vi "Trial v4.vi"(2 "error in (no error)":errorcluster, 3 "queue in":refnum<queue>, 4 "DDA":bool=TRUE) -> (0 "error out":errorcluster, 1 "queue out":refnum<queue>)   [LabVIEW 2017]
uses:
  SubVI/Global.vi
  <vilib>/Analysis/NI_AALPro.lvlib
  <vilib>/robotics/Kinematics/NI_Kinematics.lvlib
  Control/RPY.ctl
  Control/Damping.ctl
  <vilib>/Analysis/NI_AALBase.lvlib
  <vilib>/Analysis/baseanly.llb/Real Dot Product.vi
  <vilib>/Analysis/_algsub.llb/Real Vector Norm.vi
panel:
  in  "RoM (deg)":dbl=75.0 format="%#_13g"
  in  "Weber's Rule":dbl[](array[numeric])=[1.05, 1.0, 0.95]
  in  "n x(s, a)":i32=3
  in  "n x(s)":i32=3
  in  "Variable":T1
  in  "Time Target (s)":dbl=10.0
  in  "epsilon":dbl=0.1
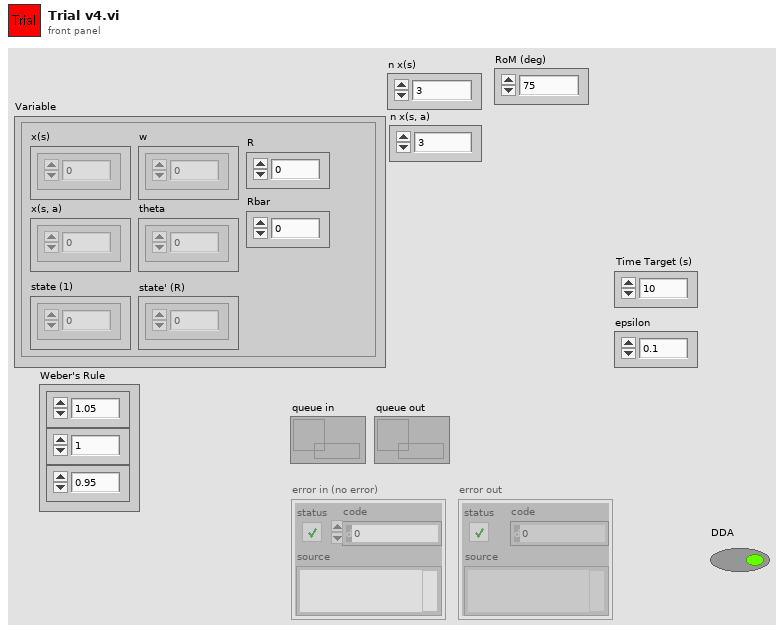
[diagram p1: front panel]
types:
  T1 = cluster{"x(s)":dbl[], "x(s, a)":dbl[], "w":dbl[], "theta":dbl[], "state (1)":dbl[], "state' (R)":dbl[], "R":dbl, "Rbar":dbl}
  T2 = typedef "RPY.ctl" = cluster{"roll":dbl, "pitch":dbl, "yaw":dbl}
  T3 = typedef "NI_Matrix.lvlib/RealMatrix.ctl" = dbl[][]
  T4 = typedef "Damping.ctl" = cluster{"Cx":dbl, "Cy":dbl, "Cz":dbl}
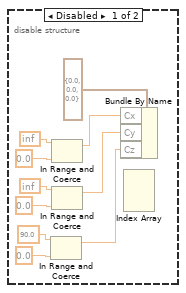
[diagram p2: hidden frame]
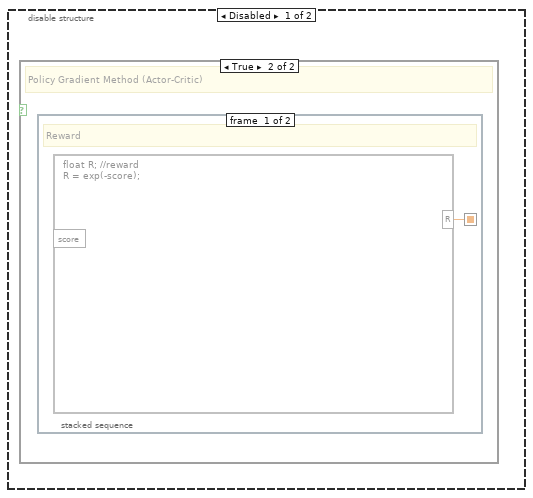
[diagram p3: hidden frame]
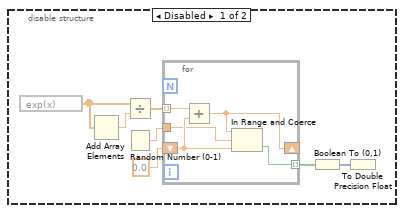
[diagram p6: hidden frame]
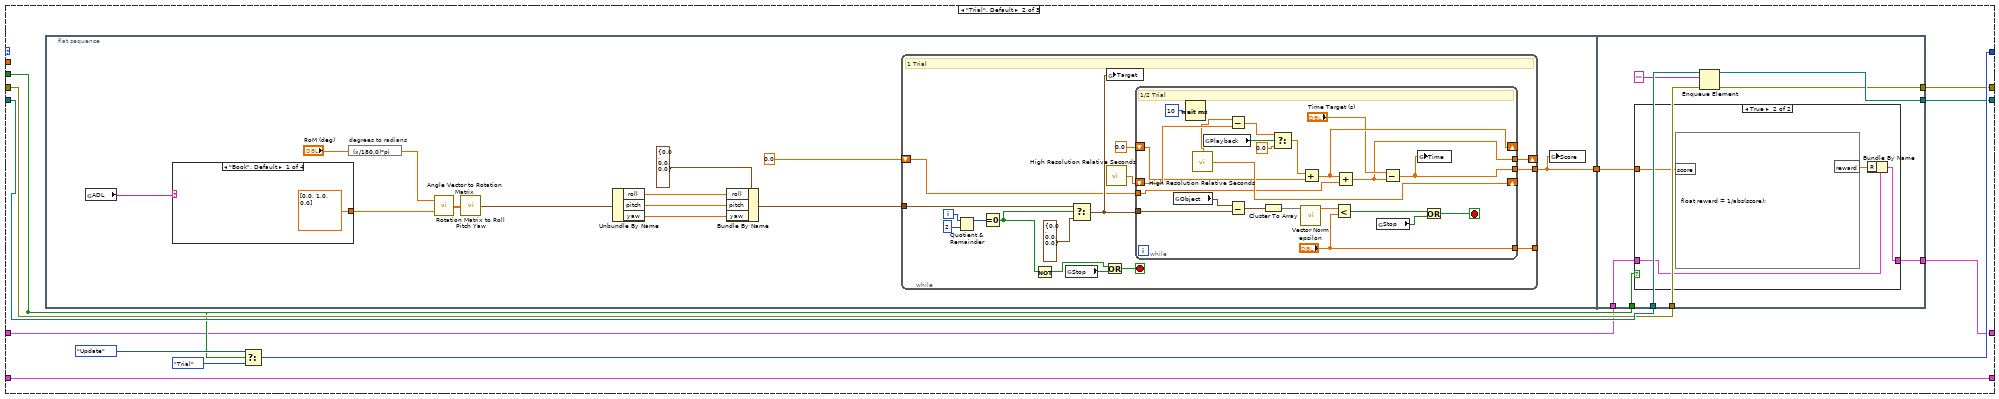
[diagram p7: hidden frame]
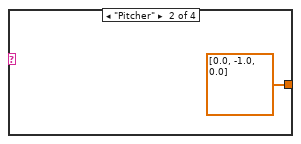
[diagram p8: hidden frame]
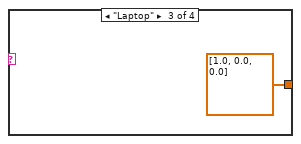
[diagram p9: hidden frame]
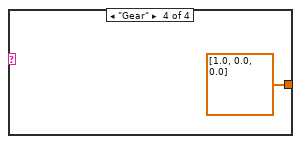
[diagram p10: hidden frame]
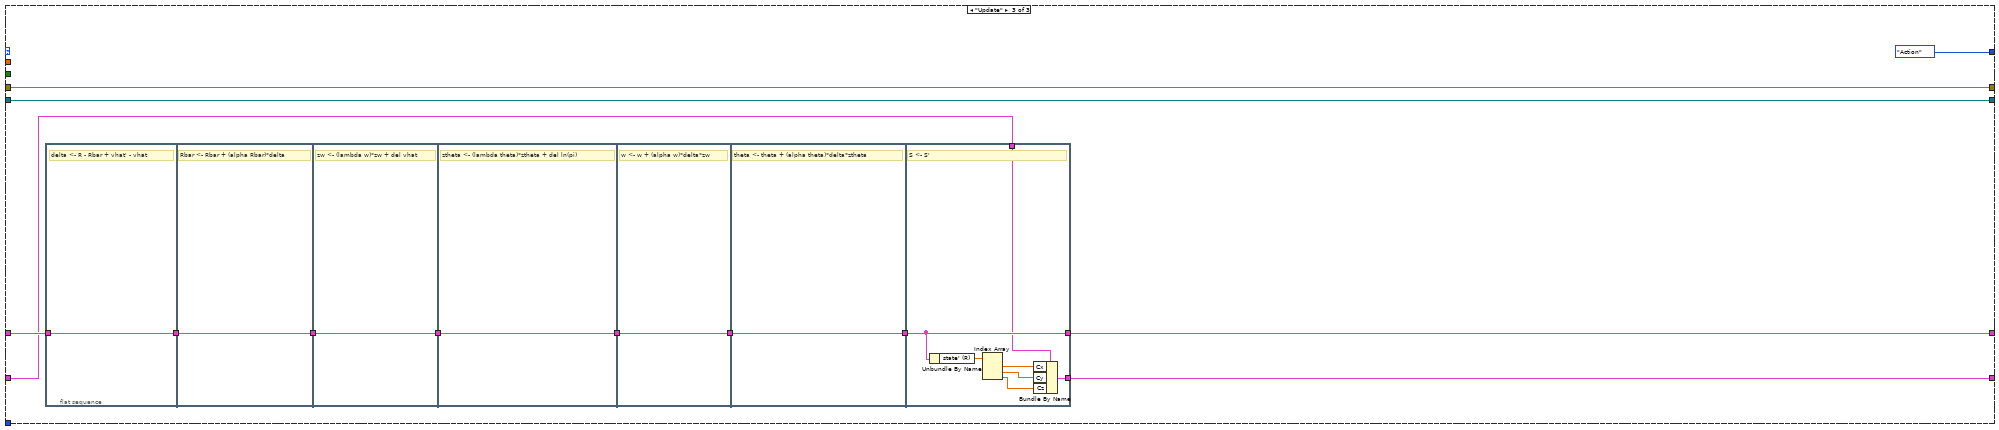
[diagram p12: hidden frame]
diagram:
  n1 = flat-sequence {
    tunnel: "error in (no error)" -> [w15]
    tunnel: "queue in" -> [w17]
    tunnel: "DDA" -> [w10]
    tunnel: [w16] -> w2
    tunnel: [w14] -> w1
    frame #0 {
      n2 = flat-sequence {
        tunnel: [w34] -> w8
        tunnel: ["n x(s, a)"] -> w7
        tunnel: [w31] -> w6
        frame #0 {
          w32 = 3
          n3 = for {
            N: w32 -> [_]
            tunnel: [w37] -> w31 mode=concatenating
            tunnel: w32 -> [w36]
            tunnel: w32 -> [w35]
            i -> [w38]
            n4 = for {
              N: w36 -> [_]
              tunnel: w38 -> [w42]
              tunnel: [w40] -> w37 mode=concatenating
              tunnel: w35 -> [w39]
              i -> [w41]
              n5 = for {
                N: w39 -> [_]
                tunnel: w42 -> [w49]
                tunnel: w41 -> [w48]
                tunnel: [w43] -> w40 mode=indexing
                i -> [w47]
                n6 = Index Array(array="Weber's Rule", index #1=w49, index #2=w48, index #3=w47) -> (element #1=w46:dbl, element #2=w45:dbl, element #3=w44:dbl)
                n7 = Build Array(w46, w45, w44) -> (w43:dbl[])
              }
            }
          }
          n8 = call "Feature Vector State Action.vi"("n x(s, a)"="n x(s, a)", "action"=0.0, "state"=dbl[] [0.0, 0.0, 0.0]) -> ("x(s, a)"=w29:dbl[])  [unwired: 8 in]
          n9 = call "Feature Vector State.vi"("n x(s)"="n x(s)", "state"=dbl[] [0.0, 0.0, 0.0]) -> ("x(s)"=w20:dbl[])  [unwired: 9 in]
          n10 = Array Size(array=w20) -> (size(s)=w21:i32)
          n11 = Array Size(array=w29) -> (size(s)=w28:i32)
          n12 = Initialize Array(0.0 ("element"), w21) -> (w19:dbl[])
          n13 = Initialize Array(0.0 ("element"), w28) -> (w25:dbl[])
          n14 = Bundle By Name(cluster="Variable", "w"=w19, "theta"=w25) -> (w34:T1)
        }
      }
      n15 = Select(t=enum16{"Action", "Trial", "Update"}."Action", s=w10, f=enum16{"Action", "Trial", "Update"}."Trial") -> (s? t:f=w11:enum16{"Action", "Trial", "Update"})
      n16 = global read "Global.vi" "Damping"() -> (w9)
      n17 = while {
        shift-right: [w58] -> w16
        shift-left: w17 -> [w60]
        shift-right: [w57] -> w14
        shift-left: w15 -> [w59]
        shift-right: [w62] -> _
        shift-left: w11 -> [w63]
        tunnel: w10 -> [w61]
        shift-right: [w55] -> _
        shift-left: w9 -> [w56]
        shift-right: [w51] -> _
        shift-left: w8 -> [w54]
        tunnel: w7 -> [w53]
        tunnel: w6 -> [w52]
        stop <- w64 stop-if-true
        # "State Machine"
        n18 = case shown="\"Action\"" w63 {
          tunnel: [enum16{"Action", "Trial", "Update"}."Trial" w116 enum16{"Action", "Trial", "Update"}."Action"] -> w62
          tunnel: w61 -> [_ w109 _]
          tunnel: w60 -> [w84 w115 w197]
          tunnel: w59 -> [w85 w110 w198]
          tunnel: [w84 w114 w197] -> w58
          tunnel: [w85 w113 w198] -> w57
          tunnel: w56 -> [w83 w111 w188]
          tunnel: [w83 w111 w187] -> w55
          tunnel: w54 -> [w68 w108 w194]
          tunnel: w53 -> [w74 _ _]
          tunnel: w52 -> [w72 _ _]
          tunnel: [w66 w107 w189] -> w51
          frame "Action" {
            w80 = 27
            n19 = Unbundle By Name(w68) -> ("theta"=w79:dbl[])
            n20 = Cluster To Array(cluster=w83) -> (array=w70:void[])
            n21 = To Double Precision Float(number=w80) -> (double precision float=w81:dbl)
            n22 = call "Convert Domain.vi"("Direction"=enum16{"Unit", "Real"}."Unit", "Real"=w70) -> ("Unit"=w69:dbl[])  [unwired: 9 in]
            n23 = Bundle By Name(cluster=w68, "state (1)"=w69) -> (w67:T1)
            n24 = for {
              N: w80 -> [_]
              tunnel: w81 -> [w105]
              tunnel: w69 -> [w101]
              tunnel: w79 -> [w99]
              tunnel: [w98] -> w78 mode=indexing
              tunnel: w74 -> [w97]
              i -> [w104]
              n25 = To Double Precision Float(number=w104) -> (double precision float=w103:dbl)
              n26 = Divide(x=w103, y=w105) -> (x/y=w102:dbl)
              n27 = call "Feature Vector State Action.vi"("n x(s, a)"=w97, "action"=w102, "state"=w101) -> ("x(s, a)"=w100:dbl[])  [unwired: 8 in]
              n28 = call-poly <vilib>:"Dot Product.vi"("Y Vector"=w100, "X Vector"=w99) -> ("X * Y"=w98:dbl)  [unwired: 1 out]
            }
            n29 = flat-sequence {
              tunnel: w78 -> [w96]
              tunnel: [w95] -> w77
              frame #0 {
                # "Softmax"
                n30 = Exponential(1:w96) -> (0:w94:dbl[])
                n31 = Add Array Elements(numeric array=w94) -> (sum=w93:dbl)
                n32 = Divide(x=w94, y=w93) -> (x/y=w95:dbl[])
              }
            }
            n33 = Random Number (0-1)() -> (number: 0 to 1=w75:dbl)
            n34 = for {
              tunnel: w77 -> [w91] mode=indexing
              shift-right: [w89] -> _
              shift-left: 0.0 -> [w90]
              tunnel: w75 -> [w92]
              tunnel: [w87] -> w73
              i -> [w87]
              stop <- w88 stop-if-true
              n35 = Add(x=w91, y=w90) -> (x+y=w89:dbl)
              n36 = In Range and Coerce(upper limit=w89, x=w92, lower limit=w90) -> (In Range?=w88:bool)  [unwired: 1 out]
            }
            n37 = Index Array(array=w72, index (row)=w73) -> (element=w71:dbl[])  [unwired: 1 in]
            n38 = Multiply(x=w70, y=w71) -> (x*y=w65:dbl[])
            n39 = Bundle By Name(cluster=w67, "state' (R)"=w65) -> (w66:T1)
          }
          frame "Trial", Default {
            n40 = flat-sequence {
              tunnel: [w118] -> w106
              tunnel: w115 -> [w181]
              tunnel: [w180] -> w114
              tunnel: [w179] -> w113
              tunnel: w110 -> [w177]
              tunnel: w109 -> [w176]
              tunnel: [w174] -> w107
              tunnel: w108 -> [w175]
              tunnel: w106 -> [w173]
              frame #0 {
                n41 = global read "Global.vi" "ADL"() -> (w122:string)
                n42 = case shown="\"Book\", Default" w122 {
                  tunnel: [dbl[] [0.0, 1.0, 0.0] dbl[] [0.0, -1.0, 0.0] dbl[] [1.0, 0.0, 0.0] dbl[] [1.0, 0.0, 0.0]] -> w121
                  frame "Book", Default {
                  }
                  frame "Pitcher" {
                  }
                  frame "Laptop" {
                  }
                  frame "Gear" {
                  }
                }
                n43 = expression code="(x/180.0)*pi" "degrees to radians"("RoM (deg)") -> (w119:dbl)
                n44 = call <vilib>:"Angle Vector to Rotation Matrix.vi"("vector"=w121, "angle"=w119) -> ("rotation matrix"=w125:T3)
                n45 = call <vilib>:"Rotation Matrix to Roll Pitch Yaw.vi"("rotation matrix"=w125) -> ("angles"=w126:cluster{"roll":dbl, "pitch":dbl, "yaw":dbl})
                n46 = Unbundle By Name(w126) -> ("roll"=w127:dbl, "pitch"=w128:dbl, "yaw"=w129:dbl)
                n47 = Bundle By Name(cluster=T2 {"roll"=0.0, "pitch"=0.0, "yaw"=0.0} ("Target"), "roll"=w127, "pitch"=w128, "yaw"=w129) -> (w123:T2)
                n48 = while {
                  tunnel: w123 -> [w145]
                  shift-right: [w137] -> _
                  shift-left: 0.0 -> [w138]
                  tunnel: [w136] -> _
                  tunnel: [w135] -> w118
                  i -> [w148]
                  stop <- w141 stop-if-true
                  # "1 Trial"
                  n49 = Quotient & Remainder(x=w148, y=2) -> (x-y*floor(x/y)=w146:i32)  [unwired: 1 out]
                  n50 = Equal To 0?(x=w146) -> (x = 0?=w140:bool)
                  n51 = Not(x=w140) -> (.not. x?=w139:bool)
                  n52 = global read "Global.vi" "Stop"() -> (w142:bool)
                  n53 = Select(t=w145, s=w140, f=T2 {"roll"=0.0, "pitch"=0.0, "yaw"=0.0} ("Target")) -> (s? t:f=w143:T2)
                  n54 = Or(x=w139, y=w142) -> (x .or. y?=w141:bool)
                  n55 = global write "Global.vi" "Target"(w143) -> ()
                  n56 = call <vilib>:"High Resolution Relative Seconds.vi"() -> ("relative seconds"=w150:dbl)
                  n57 = while {
                    tunnel: w143 -> [w157]
                    shift-right: [w163] -> _
                    shift-left: w150 -> [w164]
                    shift-right: [w155] -> _
                    shift-left: 0.0 -> [w162]
                    tunnel: w138 -> [w156]
                    tunnel: [w153] -> w137
                    tunnel: ["epsilon"] -> w136
                    tunnel: [w151] -> w135
                    stop <- w165 stop-if-true
                    # "1/2 Trial"
                    n58 = global read "Global.vi" "Object"() -> (w170:T2)
                    n59 = Wait (ms)(milliseconds to wait=u32 10) -> ()  [unwired: 1 out]
                    n60 = call <vilib>:"High Resolution Relative Seconds.vi"() -> ("relative seconds"=w163:dbl)
                    n61 = global read "Global.vi" "Playback"() -> (w161:bool)
                    n62 = Subtract(x=w163, y=w164) -> (x-y=w160:dbl)
                    n63 = Subtract(x=w170, y=w157) -> (x-y=w171:T2)
                    n64 = Cluster To Array(cluster=w171) -> (array=w172:dbl[])
                    n65 = Select(t=w160, s=w161, f=0.0) -> (s? t:f=w159:dbl)
                    n66 = call-poly <vilib>:"Vector Norm.vi"("Input Vector"=w172) -> ("norm"=w169:dbl)  [unwired: 9 in, 1 out]
                    n67 = Add(x=w159, y=w162) -> (x+y=w155:dbl)
                    n68 = Less?(x=w169, y="epsilon") -> (x < y?=w168:bool)
                    n69 = Add(x=w155, y=w156) -> (x+y=w153:dbl)
                    n70 = global read "Global.vi" "Stop"() -> (w167:bool)
                    n71 = Subtract(x="Time Target (s)", y=w153) -> (x-y=w151:dbl)
                    n72 = global write "Global.vi" "Time"(w151) -> ()
                    n73 = Or(x=w168, y=w167) -> (x .or. y?=w165:bool)
                  }
                }
                n74 = global write "Global.vi" "Score"(w118) -> ()
              }
              frame #1 {
                n75 = case shown="True" w176 {
                  tunnel: w175 -> [w182 w185]
                  tunnel: [w182 w183] -> w174
                  tunnel: w173 -> [_ w186]
                  frame False {
                  }
                  frame True {
                    n76 = formula code="float reward = 1/abs(score);"("score"=w186) -> ("reward"=w184:dbl)
                    n77 = Bundle By Name(cluster=w185, "R"=w184) -> (w183:T1)
                  }
                }
                n78 = Enqueue Element(queue=w181, element="", error in (no error)=w177) -> (queue out=w180:refnum<queue>, error out=w179:errorcluster)  [unwired: 1 in, 1 out]
              }
            }
            n79 = Select(t=enum16{"Action", "Trial", "Update"}."Update", s=w109, f=enum16{"Action", "Trial", "Update"}."Trial") -> (s? t:f=w116:enum16{"Action", "Trial", "Update"})
          }
          frame "Update" {
            n80 = flat-sequence {
              tunnel: [w200] -> w195
              tunnel: w194 -> [w200]
              tunnel: [w201] -> w196
              tunnel: w195 -> [w201]
              tunnel: w196 -> [w202]
              tunnel: [w202] -> w192
              tunnel: [w203] -> w193
              tunnel: w192 -> [w203]
              tunnel: w193 -> [w204]
              tunnel: [w204] -> w190
              tunnel: [w205] -> w191
              tunnel: w190 -> [w205]
              tunnel: [w212] -> w189
              tunnel: w191 -> [w212]
              tunnel: w188 -> [w210]
              tunnel: [w206] -> w187
              frame #0 {
                # "delta <- R - Rbar + vhat' - vhat"
              }
              frame #1 {
                # "Rbar <- Rbar + (alpha Rbar)*delta"
              }
              frame #2 {
                # "zw <- (lambda w)*zw + del vhat"
              }
              frame #3 {
                # "ztheta <- (lambda theta)*ztheta + del ln(pi)"
              }
              frame #4 {
                # "w <- w + (alpha w)*delta*zw"
              }
              frame #5 {
                # "theta <- theta + (alpha theta)*delta*ztheta"
              }
              frame #6 {
                # "S <- S'"
                n81 = Unbundle By Name(w212) -> ("state' (R)"=w211:dbl[])
                n82 = Index Array(array=w211) -> (element #1=w209:dbl, element #2=w208:dbl, element #3=w207:dbl)  [unwired: 3 in]
                n83 = Bundle By Name(cluster=w210, "Cx"=w209, "Cy"=w208, "Cz"=w207) -> (w206:cluster{})
              }
            }
          }
        }
        n84 = global read "Global.vi" "Stop"() -> (w64:bool)
      }
    }
  }
  n85 = disable-structure shown="Enabled" {
    frame Disabled {
      n86 = In Range and Coerce(upper limit=90.0, lower limit=0.0) -> (coerced(x)=w222:dbl)  [unwired: 1 in, 1 out]
      n87 = In Range and Coerce(upper limit=inf, lower limit=0.0) -> (coerced(x)=w220:dbl)  [unwired: 1 in, 1 out]
      n88 = In Range and Coerce(upper limit=inf, lower limit=0.0) -> (coerced(x)=w221:dbl)  [unwired: 1 in, 1 out]
      n89 = Bundle By Name(cluster=T4 {"Cx"=0.0, "Cy"=0.0, "Cz"=0.0} ("State"), "Cx"=w220, "Cy"=w221, "Cz"=w222) -> ()  [unwired: 1 out]
      n90 = Index Array() -> ()  [unwired: 4 in, 3 out]
    }
    frame Enabled {
    }
  }
  n91 = disable-structure shown="Enabled" {
    frame Disabled {
      n92 = expression code="exp(x)"() -> (w225:dbl[])  [unwired: 1 in]
      n93 = Add Array Elements(numeric array=w225) -> (sum=w226:dbl)
      n94 = Divide(x=w225, y=w226) -> (x/y=w223:dbl[])
      n95 = Random Number (0-1)() -> (number: 0 to 1=w227:dbl)
      n96 = for {
        shift-right: [w233] -> _
        shift-left: 0.0 -> [w234]
        tunnel: w227 -> [w232]
        tunnel: [w231] -> w228 mode=indexing
        tunnel: w223 -> [w230] mode=indexing
        n97 = Add(x=w230, y=w234) -> (x+y=w233:dbl)
        n98 = In Range and Coerce(upper limit=w233, x=w232, lower limit=w234) -> (In Range?=w231:bool)  [unwired: 1 out]
      }
      n99 = Boolean To (0,1)(Boolean=w228) -> (0, 1=w229:i16[])
      n100 = To Double Precision Float(number=w229) -> ()  [unwired: 1 out]
    }
    frame Enabled {
    }
  }
  n101 = disable-structure shown="Enabled" {
    frame Disabled {
      n102 = case shown="True" {
        selector: _ -> [_ _]
        frame False {
        }
        frame True {
          # "Policy Gradient Method (Actor-Critic)"
          n103 = stacked-sequence {
            seq-local: [w235 _] -> [_ _]
            frame #0 {
              # "Reward"
              n104 = formula code="float R; //reward\nR = exp(-score);"() -> ("R"=w235:dbl)  [unwired: 1 in]
            }
            frame #1 {
            }
          }
        }
      }
    }
    frame Enabled {
    }
  }
  "error out" <- w1
  "queue out" <- w2
